vi "Shut down.vi"(7 "Fuel Valve Position":dbl, 8 "error in":errorcluster, 9 "Forced Draft Fan":bool, 10 "Run Interlock":bool, 11 "Shutdown":bool) -> (0 "error out":errorcluster, 3 "Boolean":bool)   [LabVIEW 2013]
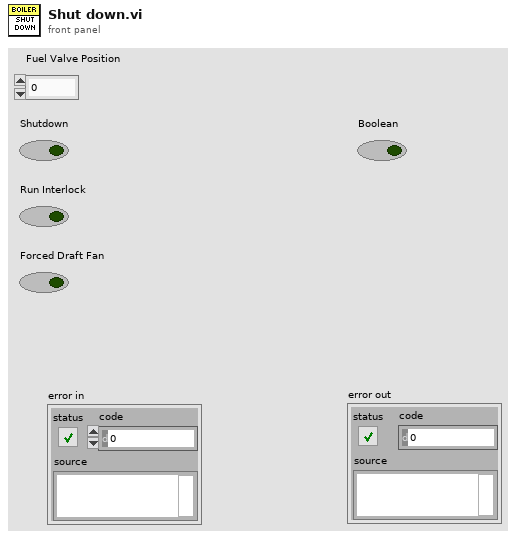
[diagram p1: front panel]
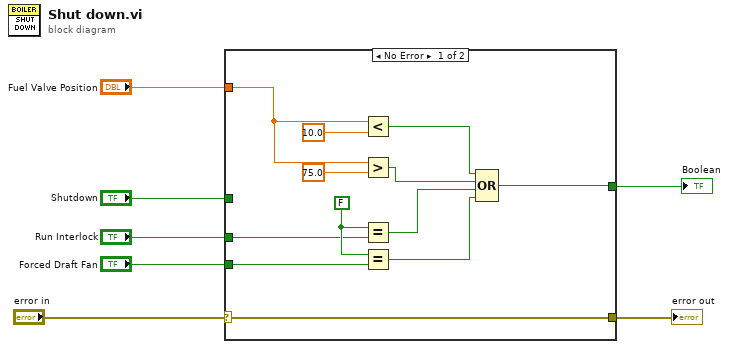
[diagram p0: block diagram]
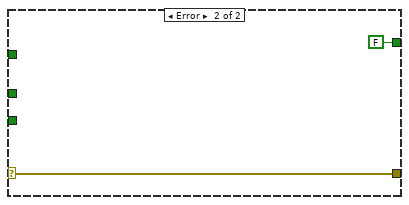
[diagram p2: hidden frame]
diagram:
  n1 = case shown="No Error" "error in" {
    selector: "error in" -> [w15 w21]
    tunnel: [w8 FALSE] -> w7
    tunnel: "Forced Draft Fan" -> [w18 _]
    tunnel: "Run Interlock" -> [w17 _]
    tunnel: "Shutdown" -> [_ _]
    tunnel: "Fuel Valve Position" -> [w16 _]
    tunnel: [w15 w21] -> w1
    frame No Error {
      w19 = FALSE ("x")
      n2 = Less?(x=w16, y=10.0) -> (x < y?=w9:bool)
      n3 = Greater?(x=w16, y=75.0) -> (0:w10:bool)
      n4 = Equal?(x=w19, y=w17) -> (x = y?=w11:bool)
      n5 = Equal?(x=w19, y=w18) -> (x = y?=w12:bool)
      n6 = Compound Arithmetic op=OR(w9, w10, w11, w12) -> (w8:bool)
    }
    frame Error {
    }
  }
  "Boolean" <- w7
  "error out" <- w1
